vi "CheckSRLinks.vi"(8 "Error In":errorcluster, 11 "SR #":string) -> (0 "Error Out":errorcluster, 1 "Documents Used (B)":bool, 3 "Documents Marked as Solution (B)":bool)   [LabVIEW 2017, in "DS_Lib.lvlib" / "SRNotesParser.lvlib"]
uses:
  SRNotesParser.lvlib
  <vilib>/httpClient/LabVIEWHTTPClient.lvlib
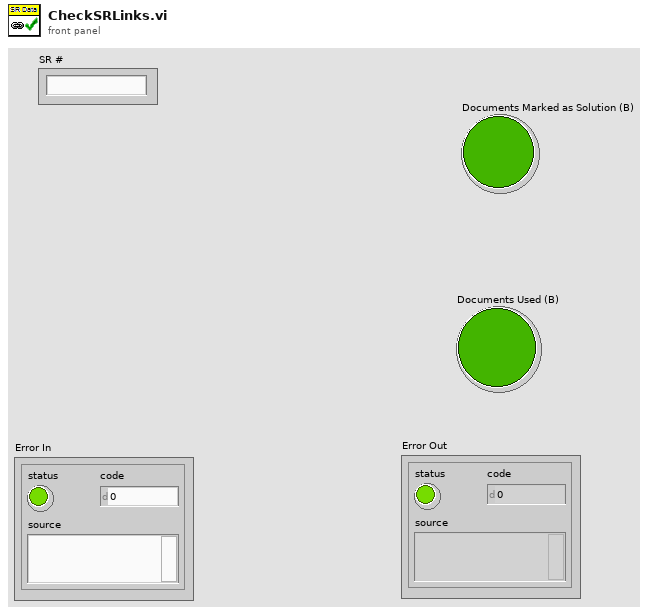
[diagram p1: front panel]
types:
  T1 = typedef "LabVIEWHTTPClient.lvlib/ClientHandle.ctl" = refnum<k1>
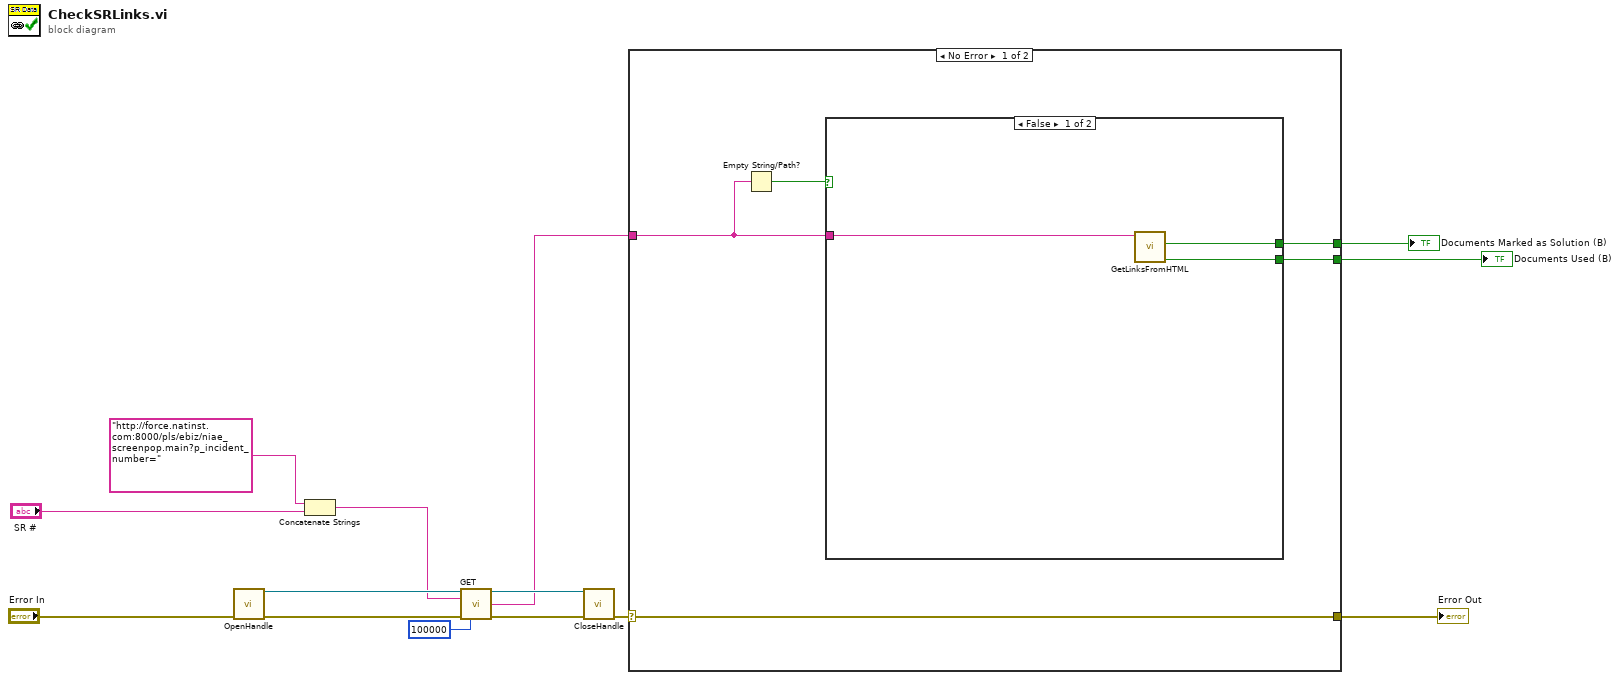
[diagram p0: block diagram]
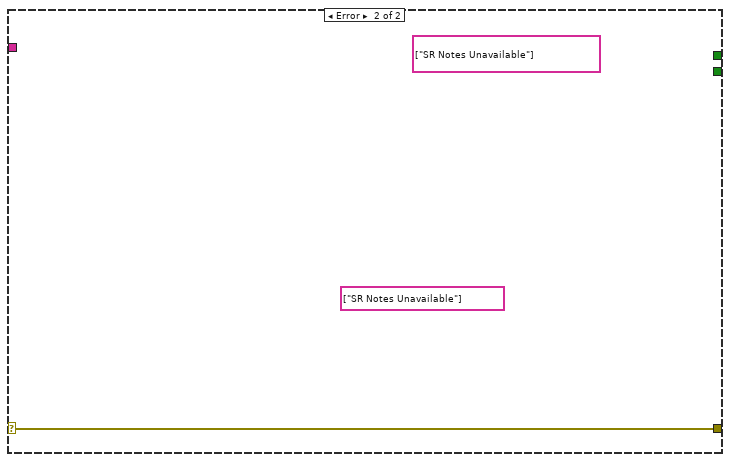
[diagram p3: hidden frame]
diagram:
  n1 = call <vilib>:"OpenHandle.vi"("error in (no error)"="Error In") -> ("client handle out"=w13:T1, "error out"=w12:errorcluster)  [unwired: 13 in]
  n2 = Concatenate Strings("http://force.natinst.com:8000/pls/ebiz/niae_screenpop.main?p_incident_number=" ("command line"), "SR #") -> (w8:string)
  n3 = call <vilib>:"GET.vi"("client handle"=w13, "url"=w8, "error in (no error)"=w12, "timeout (10000)"=100000) -> ("client handle out"=w10:T1, "body"=w6:string, "error out"=w11:errorcluster)  [unwired: 8 in, 1 out]
  n4 = call <vilib>:"CloseHandle.vi"("client handle"=w10, "error in (no error)"=w11) -> ("error out"=w4:errorcluster)  [unwired: 13 in]
  n5 = case shown="No Error" w4 {
    selector: w4 -> [w19 w23]
    tunnel: w6 -> [w17 _]
    tunnel: [w19 w23] -> w14
    tunnel: [w16 _] -> w2
    tunnel: [w15 _] -> w1
    frame No Error {
      n6 = Empty String/Path?(string/path=w17) -> (empty?=w18:bool)
      n7 = case shown="False" w18 {
        tunnel: w17 -> [w22 _]
        tunnel: [w21 _] -> w16
        tunnel: [w20 _] -> w15
        frame False {
          n8 = call "GetLinksFromHTML.vi"("SR XML in"=w22) -> ("Documents Used (B)"=w20:bool, "Documents Marked as Solution (B)"=w21:bool)  [unwired: 7 in, 2 out]
        }
        frame True {
        }
      }
    }
    frame Error {
      (unwired) string[][] [["SR Notes Unavailable"]] ("Solutions Linked")
      (unwired) string[] ["SR Notes Unavailable"] ("Array")
    }
  }
  "Error Out" <- w14
  "Documents Marked as Solution (B)" <- w2
  "Documents Used (B)" <- w1
